vi "Update_Process.vi"(0 "Car_Wash_Data_In":T1, 5 "Car_Wash_Switch_Reference":refnum<vi>, 7 "Purchase_Selection_Reference":refnum<vi>, 13 "Label.Text":string) -> (4 "Car_Wash_Data_Out":T1)   [LabVIEW 2023]
doc: "Used to update the car wash machine with the process that need to be done for the purchase"
uses:
  Control/Car_Wash_Data.ctl
  Control/Stage_Data.ctl
  Control/Car_Wash_Indicators.ctl
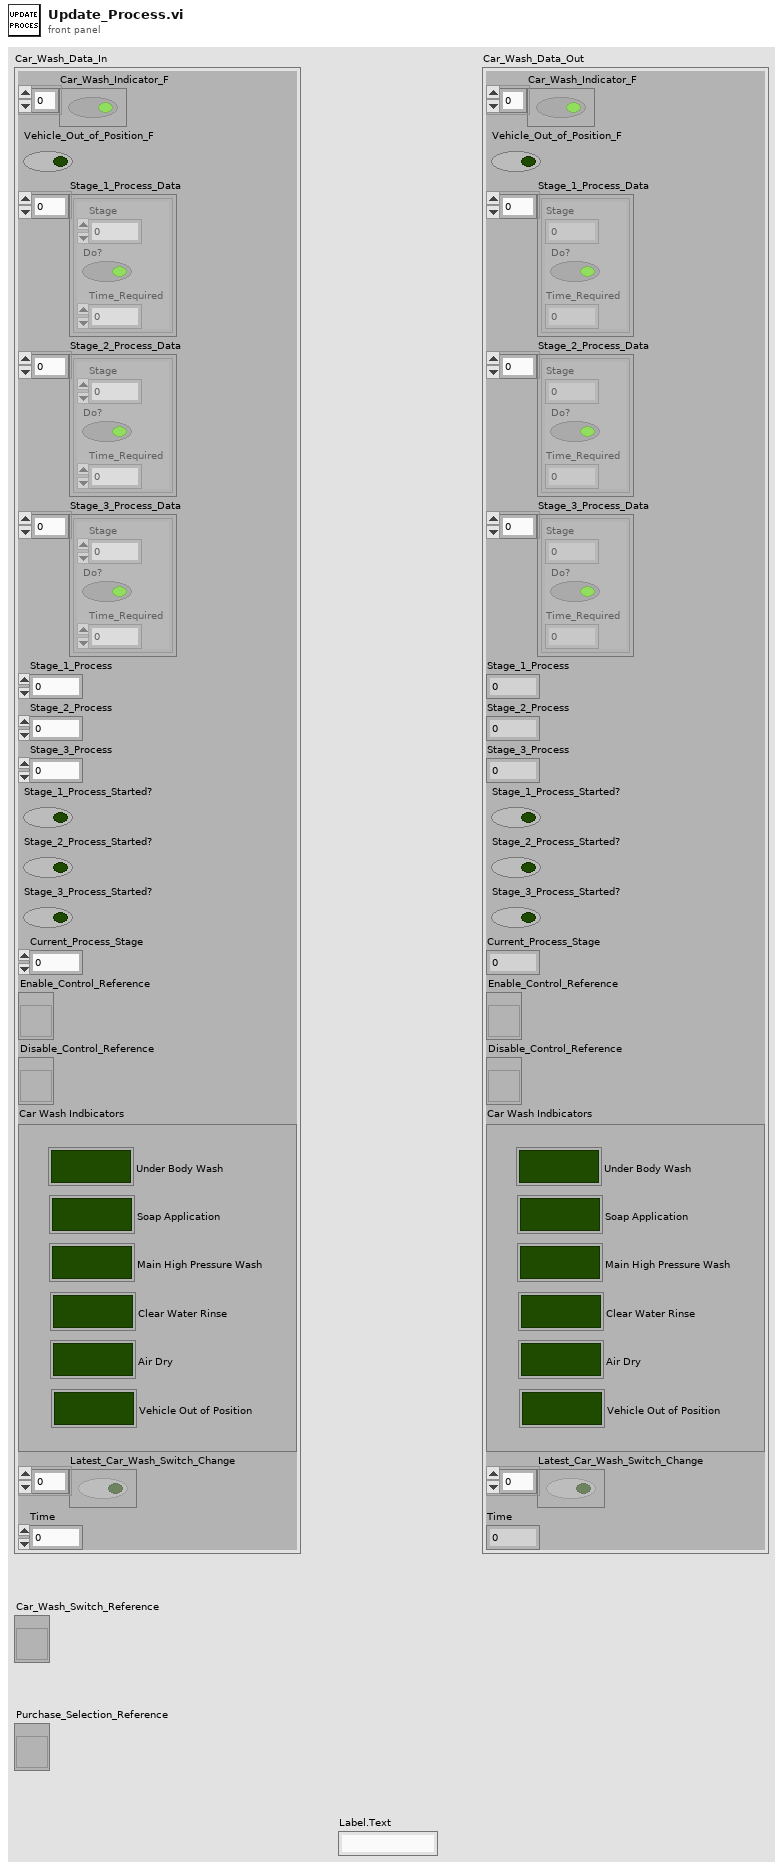
[diagram p1: front panel]
types:
  T1 = typedef "Car_Wash_Data.ctl" = cluster{"Car_Wash_Indicator_F":bool[], "Vehicle_Out_of_Position_F":bool, "Stage_1_Process_Data":T2[], "Stage_2_Process_Data":T2[], "Stage_3_Process_Data":T2[], "Stage_1_Process":i32, "Stage_2_Process":i32, "Stage_3_Process":i32, "Stage_1_Process_Started?":bool, "Stage_2_Process_Started?":bool, "Stage_3_Process_Started?":bool, "Current_Process_Stage":i32, "Enable_Control_Reference":refnum<vi>, "Disable_Control_Reference":refnum<vi>, "Car_Wash_Indicators":T3, "Latest_Car_Wash_Switch_Change":bool[], "Time":dbl}
  T2 = typedef "Stage_Data.ctl" = cluster{"Stage":i32, "Do?":bool, "Time_Required":i32}
  T3 = typedef "Car_Wash_Indicators.ctl" = cluster{"Under_Body_Wash":bool, "Soap_Application":bool, "Main_High_Pressure_Wash":bool, "Clear_Water_Rinse":bool, "Air_Dry":bool, "Vehicle_Out_of_Position":bool}
  T4 = cluster{"Stage_2_Process_Data[0]":T2, "Stage_2_Process_Data[1]":T2, "Stage_2_Process_Data[2]":T2, "Stage_2_Process_Data[3]":T2, "Stage_2_Process_Data[4]":T2, "Stage_2_Process_Data[5]":T2, "Stage_2_Process_Data[6]":T2, "Stage_2_Process_Data[7]":T2, "Stage_2_Process_Data[8]":T2}
  T5 = cluster{"Stage_3_Process_Data[0]":T2, "Stage_3_Process_Data[1]":T2, "Stage_3_Process_Data[2]":T2, "Stage_3_Process_Data[3]":T2, "Stage_3_Process_Data[4]":T2, "Stage_3_Process_Data[5]":T2, "Stage_3_Process_Data[6]":T2, "Stage_3_Process_Data[7]":T2, "Stage_3_Process_Data[8]":T2}
  T6 = cluster{"Stage_1_Process_Data[0]":T2, "Stage_1_Process_Data[1]":T2, "Stage_1_Process_Data[2]":T2, "Stage_1_Process_Data[3]":T2, "Stage_1_Process_Data[4]":T2, "Stage_1_Process_Data[5]":T2, "Stage_1_Process_Data[6]":T2, "Stage_1_Process_Data[7]":T2, "Stage_1_Process_Data[8]":T2}
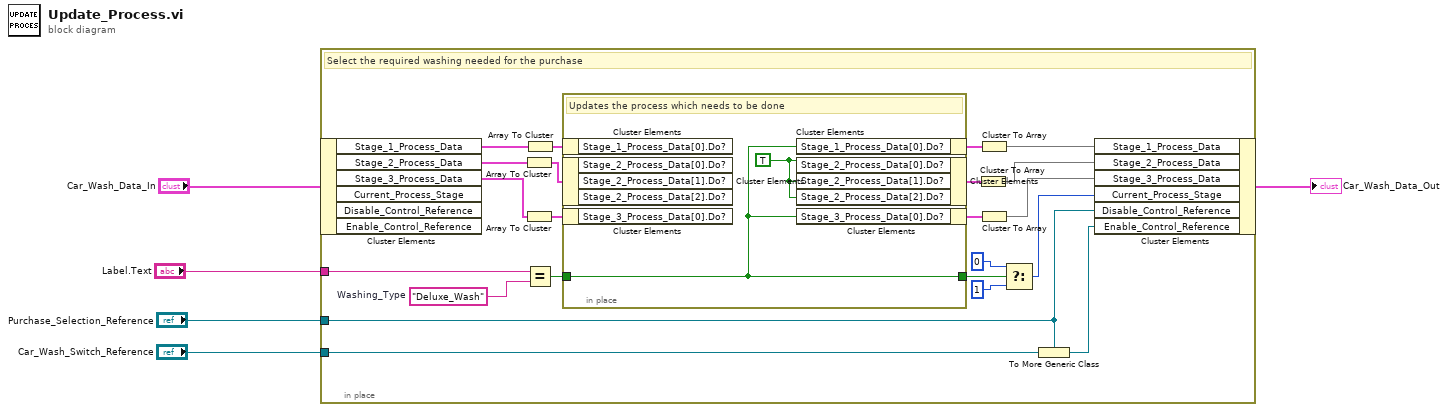
[diagram p0: block diagram]
diagram:
  n1 = in-place "In Place Element Structure" {
    in-place-border: "Label.Text" -> [w22]
    in-place-border: "Purchase_Selection_Reference" -> [w7]
    in-place-border: "Car_Wash_Switch_Reference" -> [w6]
    w23 = "Deluxe_Wash"  # Washing_Type
    # "Select the required washing needed for the purchase"
    n2 = in-place-cluster #1("Car_Wash_Data_In") -> ("Stage_1_Process_Data"=w27:T2[], "Stage_2_Process_Data"=w17:T2[], "Stage_3_Process_Data"=w15:T2[])  [unwired: 3 out]
    n3 = Array To Cluster(array=w17) -> (cluster=w16:T4)
    n4 = Array To Cluster(array=w15) -> (cluster=w14:T5)
    n5 = Array To Cluster(array=w27) -> (cluster=w26:T6)
    n6 = Equal?(x=w22, y=w23) -> (x = y?=w21:bool)
    n7 = in-place "In Place Element Structure" {
      in-place-border: w21 -> [w28]
      in-place-border: [w28] -> w20
      w29 = TRUE
      # "Updates the process which needs to be done"
      n8 = in-place-cluster #2(w26) -> ()  [unwired: 1 out]
      n9 = in-place-cluster #3(w16) -> ()  [unwired: 3 out]
      n10 = in-place-cluster #4(w14) -> ()  [unwired: 1 out]
      n11 = in-place-cluster #2("Stage_1_Process_Data[0].Do?"=w28) -> (w25:T6)
      n12 = in-place-cluster #3("Stage_2_Process_Data[0].Do?"=w29, "Stage_2_Process_Data[1].Do?"=w29, "Stage_2_Process_Data[2].Do?"=w29) -> (w13:T4)
      n13 = in-place-cluster #4("Stage_3_Process_Data[0].Do?"=w28) -> (w11:T5)
    }
    n14 = Cluster To Array(cluster=w13) -> (array=w12:T2[])
    n15 = Cluster To Array(cluster=w25) -> (array=w24:T2[])
    n16 = Cluster To Array(cluster=w11) -> (array=w10:T2[])
    n17 = Select(t=0, s=w20, f=1) -> (s? t:f=w18:i32)
    n18 = To More Generic Class(target class=w7, reference=w6) -> (generic class reference=w8:refnum<vi>)
    n19 = in-place-cluster #1("Stage_1_Process_Data"=w24, "Stage_2_Process_Data"=w12, "Stage_3_Process_Data"=w10, "Current_Process_Stage"=w18, "Disable_Control_Reference"=w7, "Enable_Control_Reference"=w8) -> (→"Car_Wash_Data_Out":T1)
  }
